vi "ConfigDevice.vi"(8 "error in (no error)":errorcluster, 11 "PacificPowerSource in":refnum<class "PacificPowerSource.lvclass">) -> (0 "error out":errorcluster, 3 "PacificPowerSource out":refnum<class "PacificPowerSource.lvclass">)   [LabVIEW 2018, in "AcPwrPlugins.lvlib" / "PacificPowerSource.lvclass"]
doc: "This VI configures the device based on the properties set in the preference dialog."
uses:
  PacificPowerSource.lvclass
  TypeDefs/ConfigDevicesModeSelection.ctl
  <instrlib>/Pacific Power UPC Series/Pacific Power UPC Series.lvlib
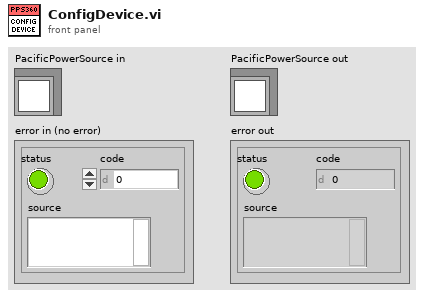
[diagram p1: front panel]
types:
  T1 = typedef "AcPwrPlugins.lvlib/PacificPowerSource.lvclass/ConfigDevicesModeSelection.ctl" = enum16{"Error", "ConfigureOutput", "VoltageLimit", "VoltageRange", "InitialVoltage", "FrequencyLimits", "FrequencyRange", "Impedance", "Waveform", "CustomWaveform", "Execute Program", "EnableOutput"}
  T2 = typedef "AcPwrPlugins.lvlib/PacificPowerSource.lvclass/Modules.ctl" = cluster{"Handle":string, "Connected":bool, "Clear Device (F)":bool, "btnIdQuery":bool, "btnReset":bool, "Program #":cluster{"Phase B (Degrees)":i32, "Waveform A (1: Sine)":i32, "Voltage Level (Va)":dbl, "Program Number (0)":i32, "Voltage Level (Vb) ":dbl, "Form (3: Three)":u16, "Coupling  (0: Direct)":u16, "Frequency (45Hz)":dbl, "Current Limit (40A)":dbl, "Phase C (Degrees)":i32, "Voltage Level (Vc)":dbl, "Waveform B (1: Sine)":i32, "Waveform C (1: Sine)":i32}[], "Impedance Parameters (off, 0.00)":cluster{"State":bool, "Impedance":dbl}, "Transient Execution (F)":bool, "OutputEnabled":bool, "Source Range":cluster{"Frequency Minimum (45 Hz)":dbl, "Frequency Maximum (1200 Hz)":dbl, "Voltage Maximum (V)":dbl, "Voltage Minimum (V)":dbl, "Range Control (0: Auto)":u16, "Initial Voltage (0V)":u16, "Frequency Range (600Hz)":u16}, "Port Type":enum16{"GPIB", "Serial"}}[]
  T3 = cluster{"Phase B (Degrees)":i32, "Waveform A (1: Sine)":i32, "Voltage Level (Va)":dbl, "Program Number (0)":i32, "Voltage Level (Vb) ":dbl, "Form (3: Three)":u16, "Coupling  (0: Direct)":u16, "Frequency (45Hz)":dbl, "Current Limit (40A)":dbl, "Phase C (Degrees)":i32, "Voltage Level (Vc)":dbl, "Waveform B (1: Sine)":i32, "Waveform C (1: Sine)":i32}[]
  T4 = cluster{"Phase B (Degrees)":i32, "Waveform A (1: Sine)":i32, "Voltage Level (Va)":dbl, "Program Number (0)":i32, "Voltage Level (Vb) ":dbl, "Form (3: Three)":u16, "Coupling  (0: Direct)":u16, "Frequency (45Hz)":dbl, "Current Limit (40A)":dbl, "Phase C (Degrees)":i32, "Voltage Level (Vc)":dbl, "Waveform B (1: Sine)":i32, "Waveform C (1: Sine)":i32}
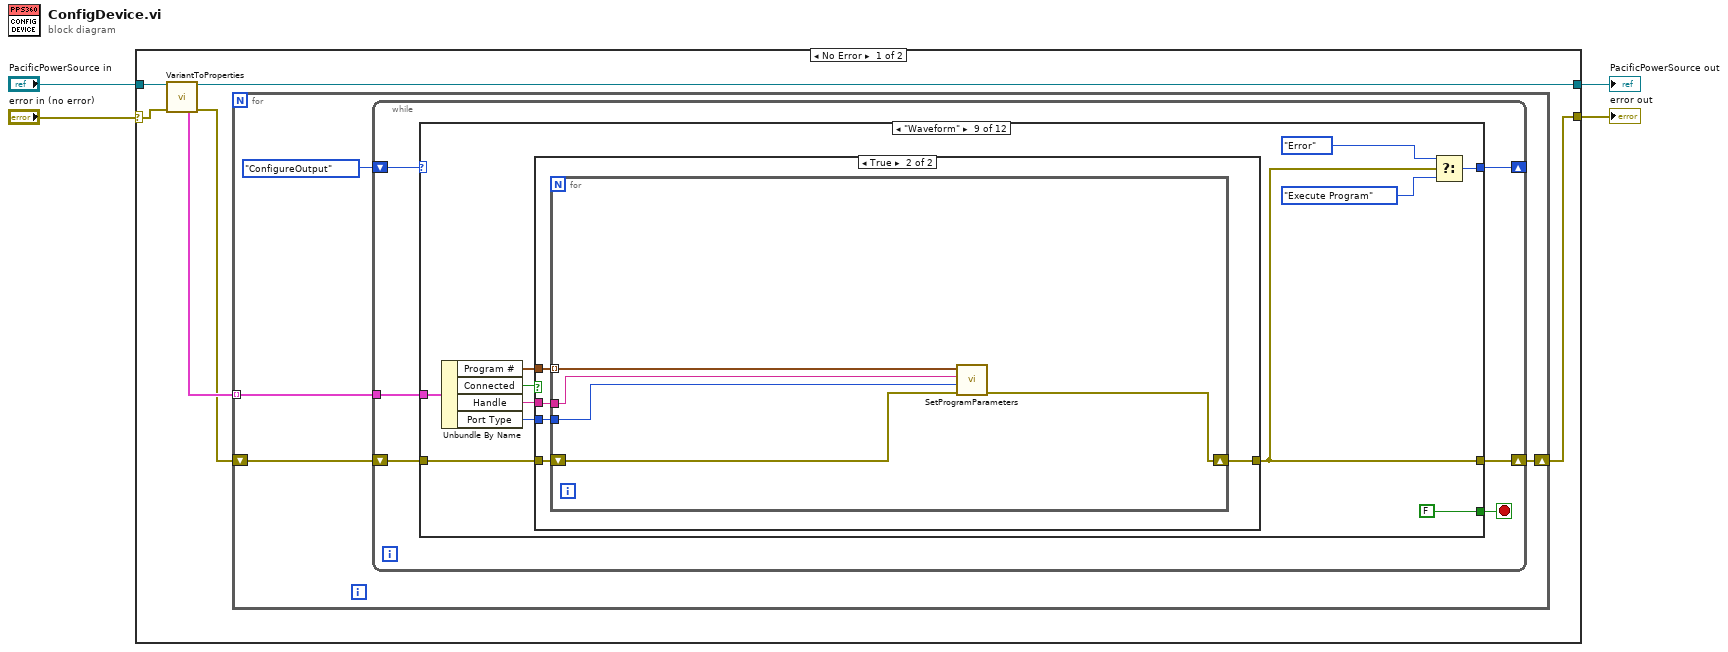
[diagram p0: block diagram]
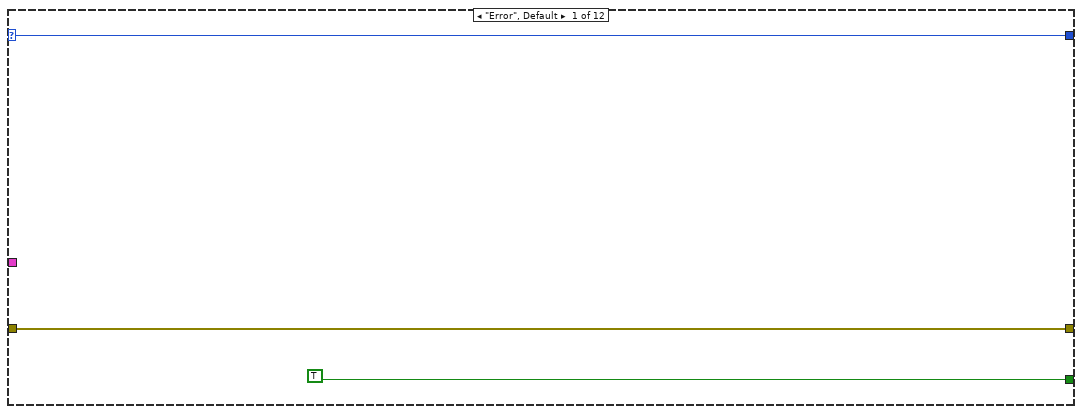
[diagram p2: hidden frame]
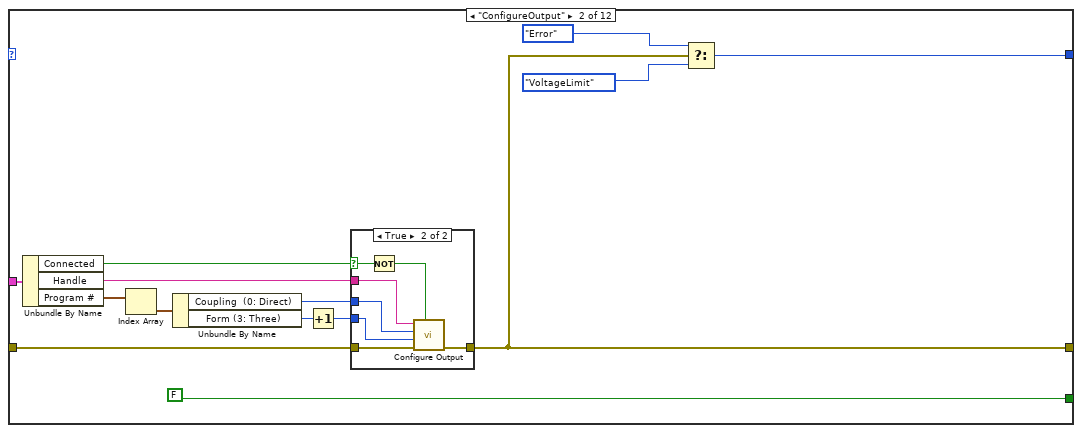
[diagram p3: hidden frame]
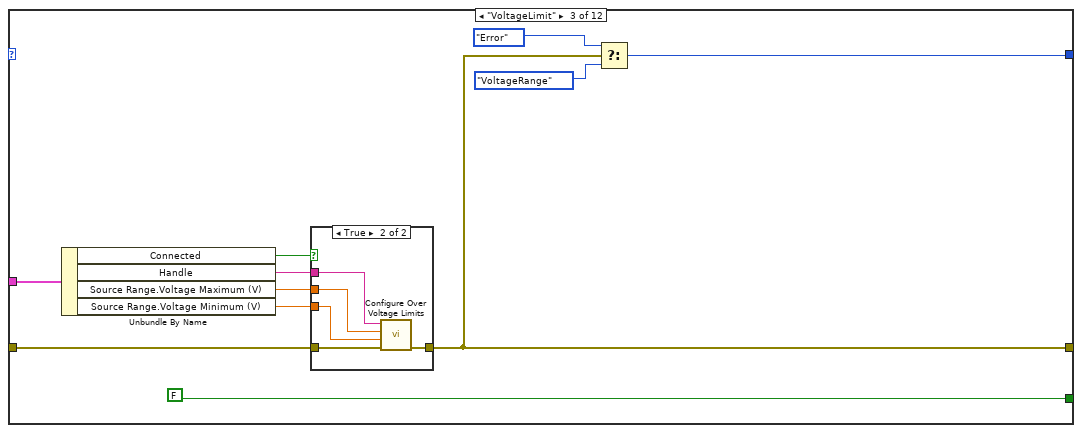
[diagram p5: hidden frame]
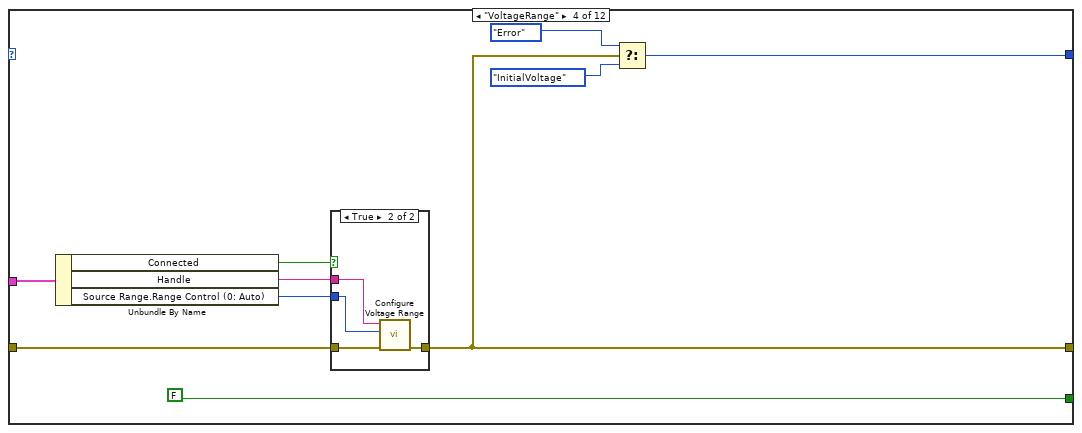
[diagram p7: hidden frame]
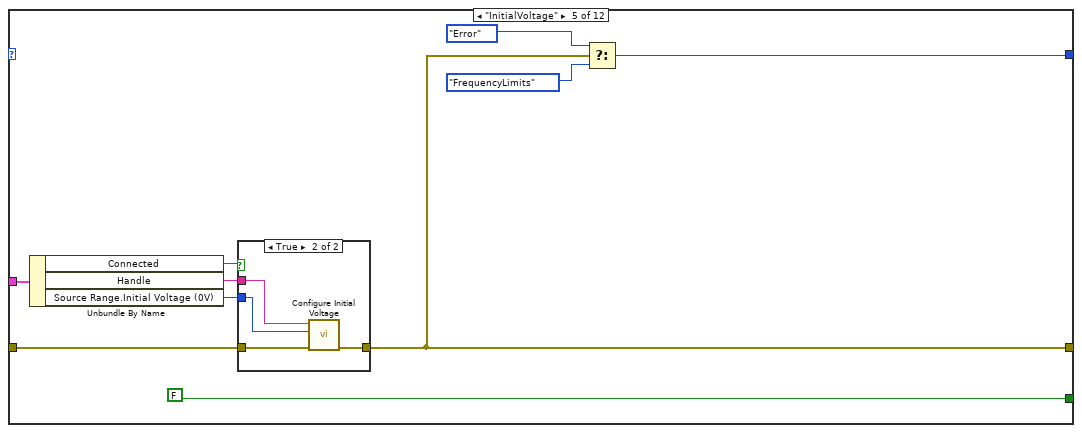
[diagram p9: hidden frame]
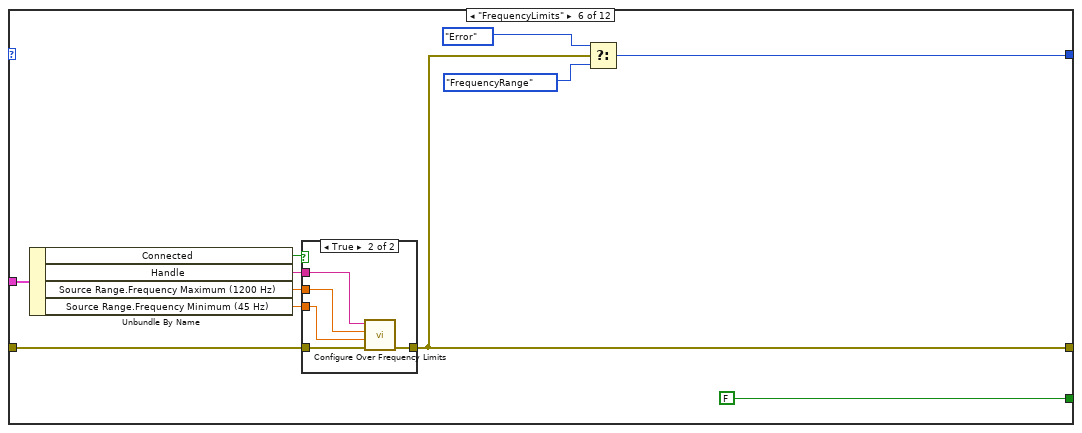
[diagram p11: hidden frame]
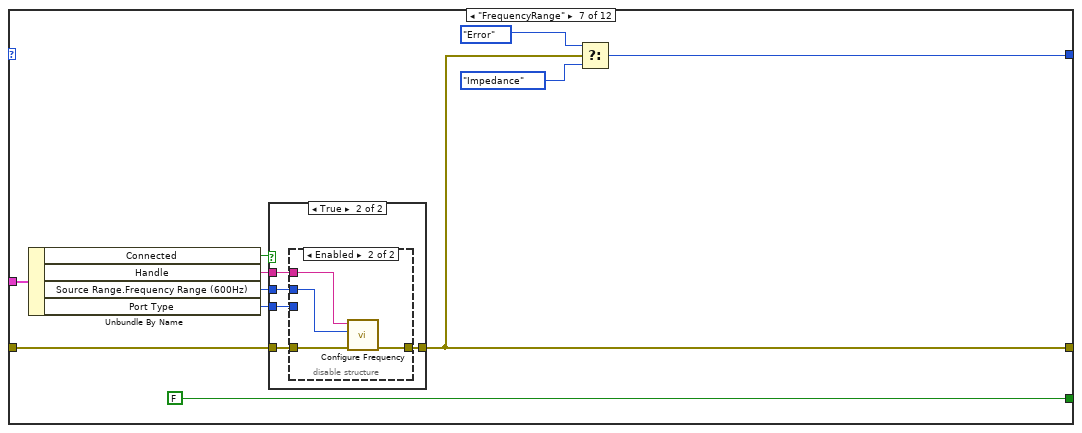
[diagram p13: hidden frame]
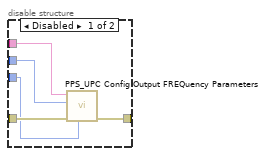
[diagram p15: hidden frame]
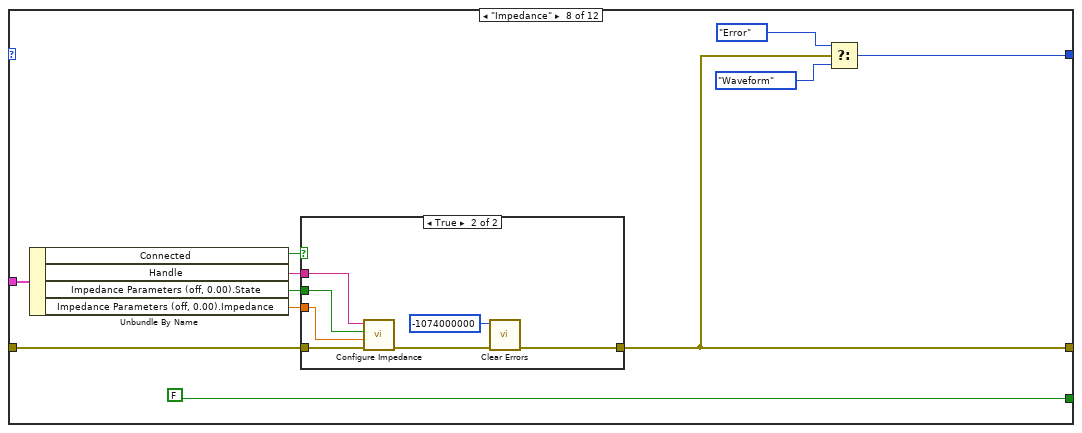
[diagram p16: hidden frame]
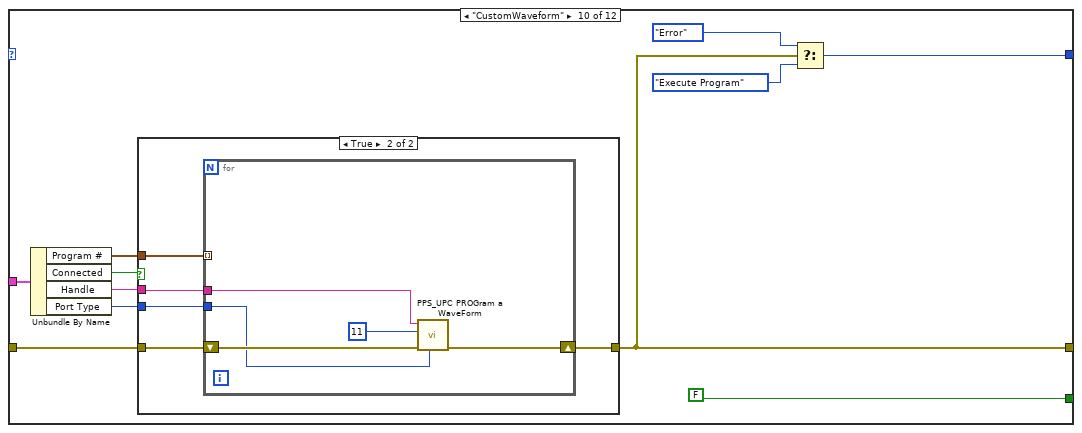
[diagram p19: hidden frame]
diagram:
  n1 = case shown="No Error" "error in (no error)" {
    selector: "error in (no error)" -> [w5 w242]
    tunnel: [w10 w242] -> w4
    tunnel: [w7 w241] -> w3
    tunnel: "PacificPowerSource in" -> [w6 w241]
    frame No Error {
      n2 = call "VariantToProperties.vi"("PacificPowerSource in"=w6, "error in (no error)"=w5) -> ("PacificPowerSource out"=w7:refnum<class "PacificPowerSource.lvclass">, "Modules"=w9:T2, "error out"=w8:errorcluster)  [unwired: 7 in, 4 out]
      n3 = for {
        tunnel: w9 -> [w14] mode=indexing
        shift-right: [w12] -> w10
        shift-left: w8 -> [w13]
        n4 = while {
          tunnel: w14 -> [w20]
          shift-right: [w18] -> w12
          shift-left: w13 -> [w19]
          shift-right: [w15] -> _
          shift-left: ConfigDevicesModeSelection."ConfigureOutput" ("Enum") -> [w17]
          stop <- w16 stop-if-true
          n5 = case shown="\"Waveform\"" w17 {
            selector: w17 -> [w21 _ _ _ _ _ _ _ _ _ _ w223]
            tunnel: w20 -> [_ w31 w56 w72 w87 w103 w120 w139 w161 w183 w210 w228]
            tunnel: w19 -> [w23 w35 w53 w69 w83 w98 w116 w143 w163 w185 w211 w231]
            tunnel: [w23 w33 w51 w67 w81 w96 w114 w141 w156 w178 w208 w229] -> w18
            tunnel: [TRUE FALSE FALSE FALSE FALSE FALSE FALSE FALSE FALSE FALSE w199 TRUE] -> w16
            tunnel: [w21 w32 w50 w66 w80 w95 w113 w140 w157 w179 w206 w223] -> w15
            frame "Error", Default {
            }
            frame "ConfigureOutput" {
              n6 = Unbundle By Name(w31) -> ("Connected"=w37:bool, "Handle"=w36:string, "Program #"=w28:T3)
              n7 = Index Array(array=w28) -> (element=w27:T4)  [unwired: 1 in]
              n8 = Unbundle By Name(w27) -> ("Coupling  (0: Direct)"=w26:u16, "Form (3: Three)"=w25:u16)
              n9 = Increment(x=w25) -> (x+1=w24:u16)
              n10 = case shown="True" w37 {
                selector: w37 -> [_ w41]
                tunnel: w36 -> [_ w43]
                tunnel: w35 -> [w38 w44]
                tunnel: [w38 w45] -> w33
                tunnel: w26 -> [_ w42]
                tunnel: w24 -> [_ w39]
                frame False {
                }
                frame True {
                  n11 = Not(x=w41) -> (.not. x?=w40:bool)
                  n12 = call <instrlib>:"Configure Output.vi"("Enable Output (T: Enable)"=w40, "error in (no error)"=w44, "Form (3: Three)"=w39, "Coupling  (0: Direct)"=w42, "VISA resource name"=w43) -> ("error out"=w45:errorcluster)  [unwired: 5 in, 1 out]
                }
              }
              n13 = Select(t=ConfigDevicesModeSelection."Error" ("Enum"), s=w33, f=ConfigDevicesModeSelection."VoltageLimit" ("Enum")) -> (s? t:f=w32:T1)
            }
            frame "VoltageLimit" {
              n14 = Unbundle By Name(w56) -> ("Connected"=w49:bool, "Handle"=w55:string, "Source Range.Voltage Maximum (V)"=w54:dbl, "Source Range.Voltage Minimum (V)"=w48:dbl)
              n15 = case shown="True" w49 {
                tunnel: w55 -> [_ w60]
                tunnel: w54 -> [_ w59]
                tunnel: w53 -> [w57 w62]
                tunnel: [w57 w61] -> w51
                tunnel: w48 -> [_ w58]
                frame False {
                }
                frame True {
                  n16 = call <instrlib>:"Configure Over Voltage Limits.vi"("error in (no error)"=w62, "Low Limit (0.0 V)"=w58, "High Limit (600.0 V)"=w59, "VISA resource name"=w60) -> ("error out"=w61:errorcluster)  [unwired: 6 in, 1 out]
                }
              }
              n17 = Select(t=ConfigDevicesModeSelection."Error" ("Enum"), s=w51, f=ConfigDevicesModeSelection."VoltageRange" ("Enum")) -> (s? t:f=w50:T1)
            }
            frame "VoltageRange" {
              n18 = Unbundle By Name(w72) -> ("Connected"=w65:bool, "Handle"=w71:string, "Source Range.Range Control (0: Auto)"=w70:u16)
              n19 = case shown="True" w65 {
                tunnel: w71 -> [_ w75]
                tunnel: w70 -> [_ w74]
                tunnel: w69 -> [w73 w77]
                tunnel: [w73 w76] -> w67
                frame False {
                }
                frame True {
                  n20 = call <instrlib>:"Configure Voltage Range.vi"("error in (no error)"=w77, "Range Control (0: Auto)"=w74, "VISA resource name"=w75) -> ("error out"=w76:errorcluster)  [unwired: 7 in, 1 out]
                }
              }
              n21 = Select(t=ConfigDevicesModeSelection."Error" ("Enum"), s=w67, f=ConfigDevicesModeSelection."InitialVoltage" ("Enum")) -> (s? t:f=w66:T1)
            }
            frame "InitialVoltage" {
              n22 = Unbundle By Name(w87) -> ("Connected"=w86:bool, "Handle"=w85:string, "Source Range.Initial Voltage (0V)"=w84:u16)
              n23 = case shown="True" w86 {
                tunnel: w85 -> [_ w90]
                tunnel: w84 -> [_ w89]
                tunnel: w83 -> [w88 w91]
                tunnel: [w88 w92] -> w81
                frame False {
                }
                frame True {
                  n24 = call <instrlib>:"Configure Initial Voltage.vi"("error in (no error)"=w91, "Initial Voltage (0: 0 V)"=w89, "VISA resource name"=w90) -> ("error out"=w92:errorcluster)  [unwired: 7 in, 1 out]
                }
              }
              n25 = Select(t=ConfigDevicesModeSelection."Error" ("Enum"), s=w81, f=ConfigDevicesModeSelection."FrequencyLimits" ("Enum")) -> (s? t:f=w80:T1)
            }
            frame "FrequencyLimits" {
              n26 = Unbundle By Name(w103) -> ("Connected"=w102:bool, "Handle"=w101:string, "Source Range.Frequency Maximum (1200 Hz)"=w100:dbl, "Source Range.Frequency Minimum (45 Hz)"=w99:dbl)
              n27 = case shown="True" w102 {
                tunnel: w101 -> [_ w107]
                tunnel: w100 -> [_ w106]
                tunnel: w99 -> [_ w105]
                tunnel: w98 -> [w104 w108]
                tunnel: [w104 w109] -> w96
                frame False {
                }
                frame True {
                  n28 = call <instrlib>:"Configure Over Frequency Limits.vi"("error in (no error)"=w108, "Low Limit (45.0 Hz)"=w105, "High Limit (1200.0 Hz)"=w106, "VISA resource name"=w107) -> ("error out"=w109:errorcluster)  [unwired: 6 in, 1 out]
                }
              }
              n29 = Select(t=ConfigDevicesModeSelection."Error" ("Enum"), s=w96, f=ConfigDevicesModeSelection."FrequencyRange" ("Enum")) -> (s? t:f=w95:T1)
            }
            frame "FrequencyRange" {
              n30 = Unbundle By Name(w120) -> ("Connected"=w119:bool, "Handle"=w118:string, "Source Range.Frequency Range (600Hz)"=w117:u16, "Port Type"=w110:enum16{"GPIB", "Serial"})
              n31 = case shown="True" w119 {
                tunnel: w118 -> [_ w122]
                tunnel: w117 -> [_ w124]
                tunnel: w116 -> [w121 w125]
                tunnel: [w121 w126] -> w114
                tunnel: w110 -> [_ w123]
                frame False {
                }
                frame True {
                  n32 = disable-structure shown="Enabled" {
                    disable-tunnel: [w131 w134] -> w126
                    disable-tunnel: w125 -> [w130 w135]
                    disable-tunnel: w124 -> [w129 w132]
                    disable-tunnel: w123 -> [w128 _]
                    disable-tunnel: w122 -> [w127 w133]
                    frame Disabled {
                      n33 = call <instrlib>:"PPS_UPC Config Output FREQuency Parameters.vi"("Port Type"=w128, "error in (no error)"=w130, "Frequency Span (600)"=w129, "VISA session"=w127) -> ("error out"=w131:errorcluster)  [unwired: 6 in, 1 out]
                    }
                    frame Enabled {
                      n34 = call <instrlib>:"Configure Frequency.vi"("error in (no error)"=w135, "Frequency Range (600 Hz)"=w132, "VISA resource name"=w133) -> ("error out"=w134:errorcluster)  [unwired: 7 in, 1 out]
                    }
                  }
                }
              }
              n35 = Select(t=ConfigDevicesModeSelection."Error" ("Enum"), s=w114, f=ConfigDevicesModeSelection."Impedance" ("Enum")) -> (s? t:f=w113:T1)
            }
            frame "Impedance" {
              n36 = Unbundle By Name(w139) -> ("Connected"=w146:bool, "Handle"=w145:string, "Impedance Parameters (off, 0.00).State"=w144:bool, "Impedance Parameters (off, 0.00).Impedance"=w138:dbl)
              n37 = case shown="True" w146 {
                tunnel: w145 -> [_ w152]
                tunnel: w144 -> [_ w151]
                tunnel: w143 -> [w147 w153]
                tunnel: [w147 w149] -> w141
                tunnel: w138 -> [_ w150]
                frame False {
                }
                frame True {
                  n38 = call <instrlib>:"Configure Impedance.vi"("error in (no error)"=w153, "Output Impedance (0.0 Ohm)"=w150, "Enable Impedance (T: Enable)"=w151, "VISA resource name"=w152) -> ("error out"=w154:errorcluster)  [unwired: 6 in, 1 out]
                  n39 = call <vilib>:"Clear Errors.vi"("error in (no error)"=w154, "specific error code to clear (0: all)"=-1074000000) -> ("error out"=w149:errorcluster)  [unwired: 4 in, 1 out]
                }
              }
              n40 = Select(t=ConfigDevicesModeSelection."Error" ("Enum"), s=w141, f=ConfigDevicesModeSelection."Waveform" ("Enum")) -> (s? t:f=w140:T1)
            }
            frame "Waveform" {
              n41 = Unbundle By Name(w161) -> ("Program #"=w160:T3, "Connected"=w165:bool, "Handle"=w164:string, "Port Type"=w155:enum16{"GPIB", "Serial"})
              n42 = case shown="True" w165 {
                tunnel: w164 -> [_ w169]
                tunnel: w163 -> [w166 w170]
                tunnel: [w166 w171] -> w156
                tunnel: w160 -> [_ w168]
                tunnel: w155 -> [_ w167]
                frame False {
                }
                frame True {
                  n43 = for {
                    shift-right: [w175] -> w171
                    shift-left: w170 -> [w176]
                    tunnel: w169 -> [w174]
                    tunnel: w168 -> [w173] mode=indexing
                    tunnel: w167 -> [w172]
                    n44 = call "SetProgramParameters.vi"("error in (no error)"=w176, "Port Type"=w172, "Handle"=w174, "Waveform"=w173) -> ("error out"=w175:errorcluster)  [unwired: 7 in]
                  }
                }
              }
              n45 = Select(t=ConfigDevicesModeSelection."Error" ("Enum"), s=w156, f=ConfigDevicesModeSelection."Execute Program" ("Enum")) -> (s? t:f=w157:T1)
            }
            frame "CustomWaveform" {
              n46 = Unbundle By Name(w183) -> ("Program #"=w182:T3, "Connected"=w187:bool, "Handle"=w186:string, "Port Type"=w177:enum16{"GPIB", "Serial"})
              n47 = case shown="True" w187 {
                tunnel: w186 -> [_ w191]
                tunnel: w185 -> [w188 w192]
                tunnel: [w188 w193] -> w178
                tunnel: w182 -> [_ w190]
                tunnel: w177 -> [_ w189]
                frame False {
                }
                frame True {
                  n48 = for {
                    shift-right: [w196] -> w193
                    shift-left: w192 -> [w198]
                    tunnel: w191 -> [w197]
                    tunnel: w190 -> [_] mode=indexing
                    tunnel: w189 -> [w194]
                    n49 = call <instrlib>:"PPS_UPC PROGram a WaveForm.vi"("Port Type"=w194, "error in (no error)"=w198, "Waveform Name"=11, "VISA session"=w197) -> ("error out"=w196:errorcluster)  [unwired: 6 in, 1 out]
                  }
                }
              }
              n50 = Select(t=ConfigDevicesModeSelection."Error" ("Enum"), s=w178, f=ConfigDevicesModeSelection."Execute Program" ("Enum")) -> (s? t:f=w179:T1)
            }
            frame "Execute Program" {
              n51 = Unbundle By Name(w210) -> ("OutputEnabled"=w201:bool, "Connected"=w213:bool, "Handle"=w212:string, "Program #"=w205:T3, "Port Type"=w202:enum16{"GPIB", "Serial"})
              n52 = Index Array(array=w205) -> (element=w204:T4)  [unwired: 1 in]
              n53 = Unbundle By Name(w204) -> ("Program Number (0)"=w203:i32)
              n54 = case shown="True" w213 {
                tunnel: w212 -> [_ w218]
                tunnel: w211 -> [w215 w221]
                tunnel: [w215 w220] -> w208
                tunnel: w203 -> [_ w219]
                tunnel: w202 -> [_ w217]
                tunnel: w201 -> [w214 w216]
                tunnel: [w214 w216] -> w200
                frame False {
                }
                frame True {
                  n55 = call <instrlib>:"PPS_UPC EXECute PROGram.vi"("Port Type"=w217, "error in (no error)"=w221, "Program Name (1)"=w219, "VISA session"=w218) -> ("error out"=w220:errorcluster)  [unwired: 6 in, 1 out]
                }
              }
              n56 = Select(t=ConfigDevicesModeSelection."Error" ("Enum"), s=w208, f=ConfigDevicesModeSelection."EnableOutput" ("Enum")) -> (s? t:f=w206:T1)
              n57 = Not(x=w200) -> (.not. x?=w199:bool)
            }
            frame "EnableOutput" {
              n58 = Unbundle By Name(w228) -> ("Connected"=w233:bool, "Handle"=w232:string, "Program #"=w227:T3)
              n59 = Index Array(array=w227) -> (element=w226:T4)  [unwired: 1 in]
              n60 = Unbundle By Name(w226) -> ("Coupling  (0: Direct)"=w225:u16, "Form (3: Three)"=w224:u16)
              n61 = Increment(x=w224) -> (x+1=w222:u16)
              n62 = case shown="True" w233 {
                tunnel: w232 -> [_ w238]
                tunnel: w231 -> [w234 w239]
                tunnel: [w234 w240] -> w229
                tunnel: w225 -> [_ w236]
                tunnel: w222 -> [_ w235]
                frame False {
                }
                frame True {
                  n63 = call <instrlib>:"Configure Output.vi"("Enable Output (T: Enable)"=TRUE, "error in (no error)"=w239, "Form (3: Three)"=w235, "Coupling  (0: Direct)"=w236, "VISA resource name"=w238) -> ("error out"=w240:errorcluster)  [unwired: 5 in, 1 out]
                }
              }
            }
          }
        }
      }
    }
    frame Error {
    }
  }
  "error out" <- w4
  "PacificPowerSource out" <- w3
